vi "Print Report.vi"(6 "Path":path, 7 "in4 paths":path[](array[path]), 8 "error in (no error)":errorcluster, 10 "Rates":dbl[](array[numeric]), 11 "Test Info":T1[](array[typedef])) -> (0 "error out":errorcluster)   [LabVIEW 2011]
uses:
  Test Info.ctl
  <vilib>/Utility/file.llb/Write To Spreadsheet File (string).vi
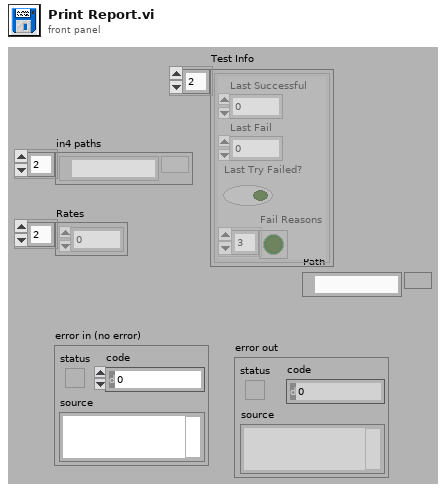
[diagram p1: front panel]
types:
  T1 = typedef "Test Info.ctl" = cluster{"Last Successful":dbl, "Last Fail":dbl, "Last Try Failed?":bool, "Fail Reasons":bool[]}
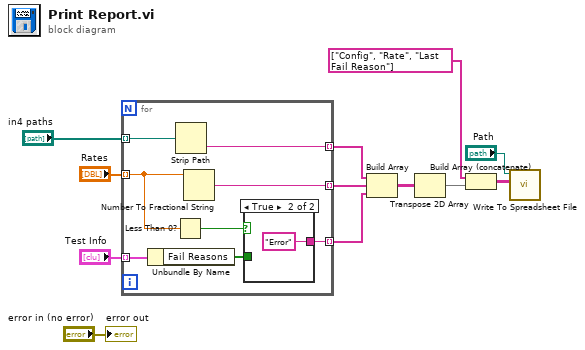
[diagram p0: block diagram]
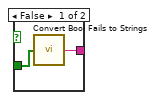
[diagram p2: hidden frame]
diagram:
  n1 = for {
    tunnel: "Rates" -> [w14] mode=indexing
    tunnel: [w20] -> w8 mode=indexing
    tunnel: "in4 paths" -> [w19] mode=indexing
    tunnel: [w18] -> w10 mode=indexing
    tunnel: "Test Info" -> [w17] mode=indexing
    tunnel: [w15] -> w5 mode=indexing
    n2 = Unbundle By Name(w17) -> ("Fail Reasons"=w16:bool[])
    n3 = Less Than 0?(x=w14) -> (x < 0?=w13:bool)
    n4 = Strip Path(path=w19) -> (name=w18:string)  [unwired: 1 out]
    n5 = Number To Fractional String(number=w14) -> (F-format string=w20:string)  [unwired: 3 in]
    n6 = case shown="True" w13 {
      tunnel: w16 -> [w22 _]
      tunnel: [w21 "Error"] -> w15
      frame False {
        n7 = call "Convert Bool Fails to Strings.vi"("Possible Failure Modes"=w22) -> ("String"=w21:string)
      }
      frame True {
      }
    }
  }
  n8 = Build Array(w10, w8, w5) -> (w9:string[][])
  n9 = Transpose 2D Array(2D array=w9) -> (transposed array=w4:string[][])
  n10 = Build Array (concatenate)(string[] ["Config", "Rate", "Last Fail Reason"], w4) -> (w3:string[][])
  n11 = call-poly <vilib>:"Write To Spreadsheet File.vi"("2D data"=w3, "file path (dialog if empty)"="Path") -> ()  [unwired: 6 in, 1 out]
  "error out" <- "error in (no error)"
